vi "Modbus_cmd.vi"(7 "Bytes to read":u32, 8 "error in (no error)":errorcluster, 9 "Data":u8[](array[numeric]), 10 "Function":u8, 11 "Serial Config":T1={"Baud"=9600, "Flow Ctl"=0, "Parity"=0, "Address"=0, "VISA resource name"=""} {"Parity" items=["None", "Odd", "Even"]; "Flow Ctl" items=["None"]; "Baud" items=["4800"=4800, "9600"=9600, "19200"=19200, "38400"=38400]}) -> (0 "error out":errorcluster, 1 "Cmd Sent":u8[](array[numeric]), 2 "Response":u8[](array[numeric]), 3 "Serial Config out":T1={"Baud"=9600, "Flow Ctl"=0, "Parity"=0, "Address"=0, "VISA resource name"=""} {"Parity" items=["None", "Odd", "Even"]; "Flow Ctl" items=["None"]; "Baud" items=["4800"=4800, "9600"=9600, "19200"=19200, "38400"=38400]})   [LabVIEW 2014, in "Omega CN9600 series.lvclass"]
uses:
  Omega CN9600 series.lvclass
  Serial_Config_Omega.ctl
  <vilib>/Instr/_visa.llb/VISA Flush IO Buffer Mask.ctl
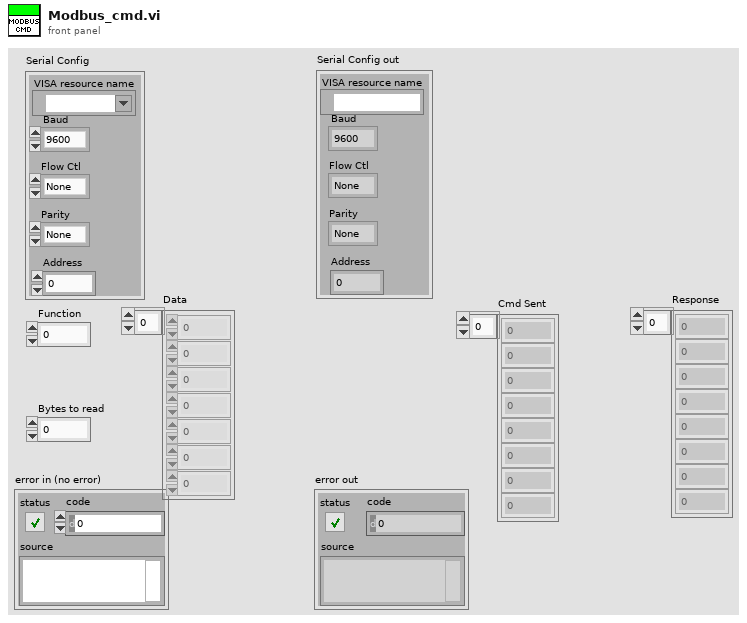
[diagram p1: front panel]
types:
  T1 = typedef "Omega CN9600 series.lvclass/Serial_Config_Omega.ctl" = cluster{"Baud":u32, "Flow Ctl":u16, "Parity":u16, "Address":u8, "VISA resource name":refnum<visa-resource-name>}
  T2 = typedef "VISA Flush IO Buffer Mask.ctl" = u16
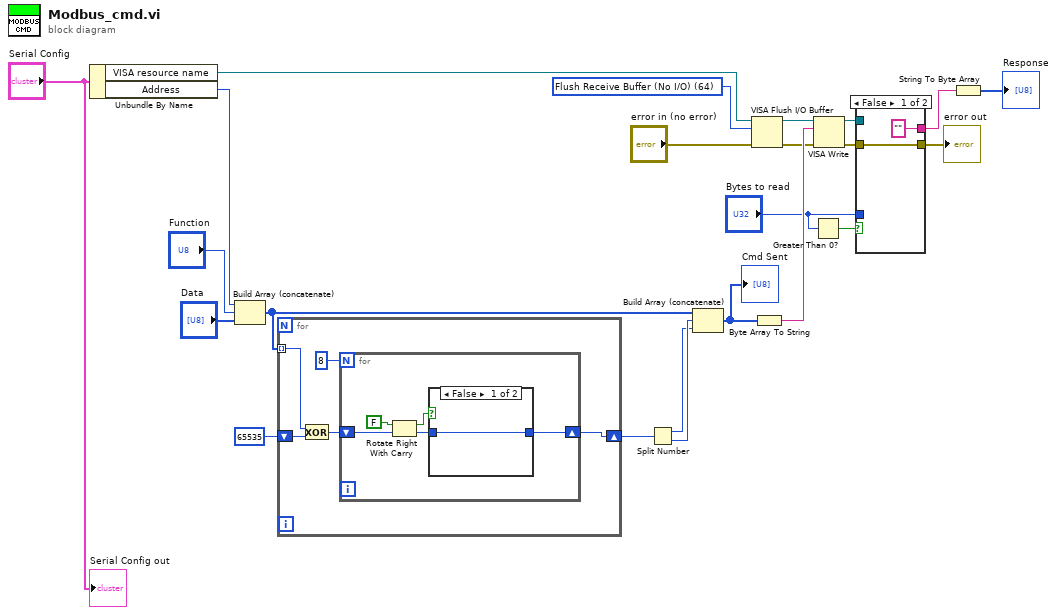
[diagram p0: block diagram]
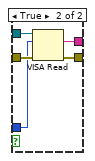
[diagram p2: hidden frame]
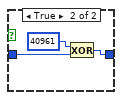
[diagram p3: hidden frame]
diagram:
  w4 = T2 64 items=["Flush Receive Buffer"=16, "Write Transmit Buffer to Device"=32, "Flush Receive Buffer (No I/O)"=64, "Flush Transmit Buffer"=128] ("Mask")
  n1 = Unbundle By Name("Serial Config") -> ("VISA resource name"=w5:refnum<visa-resource-name>, "Address"=w23:u8)
  n2 = Build Array (concatenate)(w23, "Function", "Data") -> (w18:u8[])
  n3 = for {
    shift-right: [w25] -> w17
    shift-left: u16 65535 -> [w28]
    tunnel: w18 -> [w27] mode=indexing
    n4 = Exclusive Or(1:w28, 2:w27) -> (0:w26:u16)
    n5 = for {
      N: 8 -> [_]
      shift-right: [w29] -> w25
      shift-left: w26 -> [w32]
      n6 = Rotate Right With Carry(2:w32, 3:FALSE ("carry")) -> (0:w30:u16, 1:w31:bool)
      n7 = case shown="False" w31 {
        tunnel: w30 -> [w34 w37]
        tunnel: [w34 w35] -> w29
        frame False {
        }
        frame True {
          n8 = Exclusive Or(1:w37, 2:u16 40961 ("x")) -> (0:w35:u16)
        }
      }
    }
  }
  n9 = Split Number(x=w17) -> (hi(x)=w15:u8, lo(x)=w16:u8)
  n10 = Build Array (concatenate)(w18, w16, w15) -> (w8:u8[])
  "Cmd Sent" <- w8
  n11 = VISA Flush I/O Buffer(VISA resource name=w5, mask (16)=w4, error in (no error)="error in (no error)") -> (VISA resource name out=w1:refnum<visa-resource-name>, error out=w2:errorcluster)
  n12 = Byte Array To String(unsigned byte array=w8) -> (string=w20:string)
  n13 = Greater Than 0?(x="Bytes to read") -> (x > 0?=w7:bool)
  n14 = VISA Write(VISA resource name=w1, write buffer=w20, error in (no error)=w2) -> (VISA resource name out=w13:refnum<visa-resource-name>, error out=w12:errorcluster)  [unwired: 1 out]
  n15 = case shown="False" w7 {
    tunnel: w13 -> [_ w44]
    tunnel: w12 -> [w39 w43]
    tunnel: ["" ("read buffer") w42] -> w11
    tunnel: [w39 w41] -> w9
    tunnel: "Bytes to read" -> [_ w40]
    frame False {
    }
    frame True {
      n16 = VISA Read(VISA resource name=w44, byte count=w40, error in (no error)=w43) -> (read buffer=w42:string, error out=w41:errorcluster)  [unwired: 2 out]
    }
  }
  "error out" <- w9
  n17 = String To Byte Array(string=w11) -> (unsigned byte array=→"Response":u8[])
  "Serial Config out" <- "Serial Config"
